vi "OpticsTest.vi"() -> ()   [LabVIEW 2020]
uses:
  opticstest.ctl
panel:
  in  "Case Constant\n(See Context Help)":enum16{"default"}(ring)
  in  "Boolean":bool
  in  "SeqMoveOn":bool
  in  "MoveOn":bool
  out "Options":enum16{"SequenceShot", "SingleShot", "default"}(ring)
  in  "seq":bool
  in  "single":bool
  out "State":enum16{"init", "standby", "loopy", "out"}(ring)
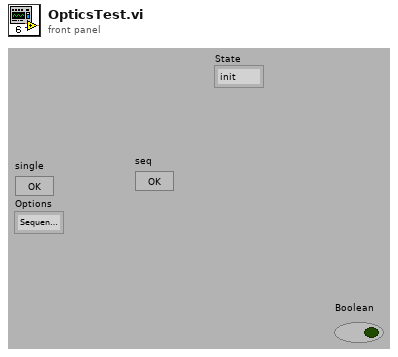
[diagram p1: front panel]
types:
  T1 = typedef "opticstest.ctl" = enum16{"_Quit_", "Init", "Ready", "CCD_shot", "HTL"}
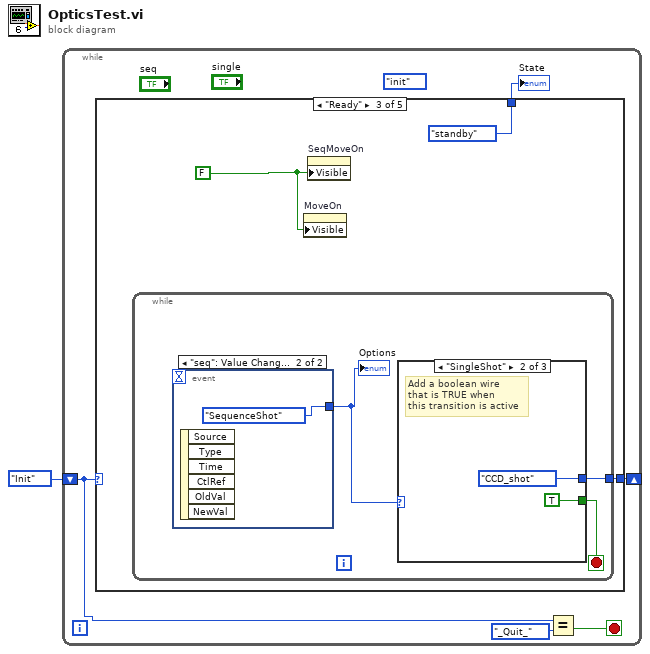
[diagram p0: block diagram]
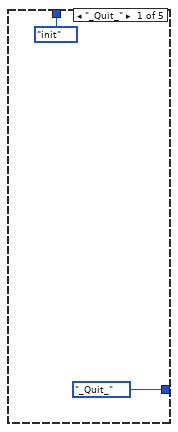
[diagram p2: hidden frame]
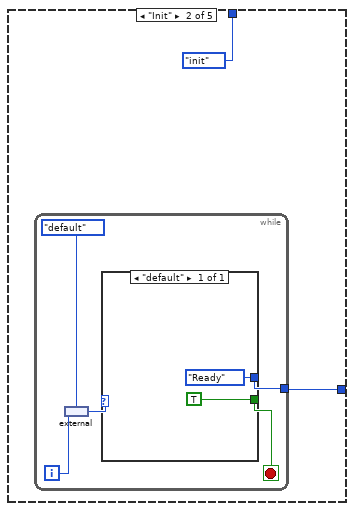
[diagram p3: hidden frame]
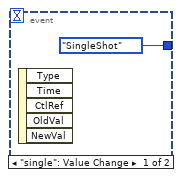
[diagram p4: hidden frame]
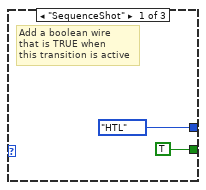
[diagram p5: hidden frame]
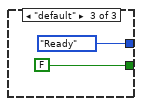
[diagram p6: hidden frame]
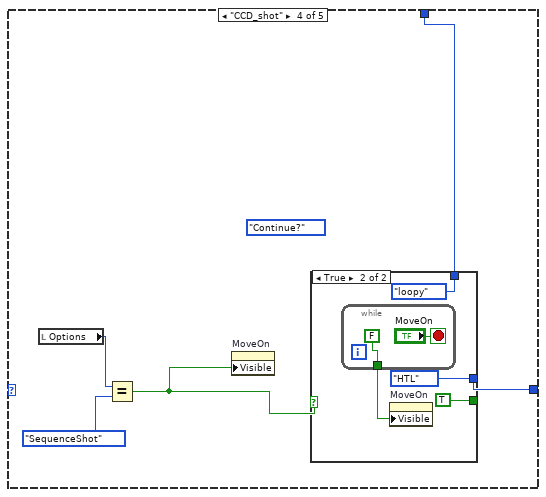
[diagram p7: hidden frame]
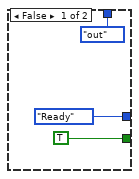
[diagram p8: hidden frame]
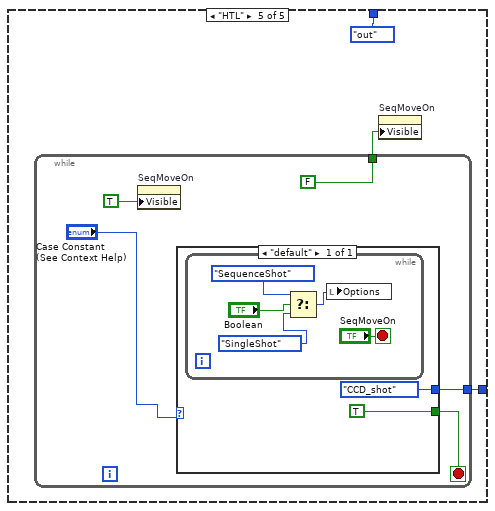
[diagram p9: hidden frame]
diagram:
  n1 = while {
    shift-right: [w5] -> _
    shift-left: opticstest."Init" -> [w6]
    stop <- w4 stop-if-true
    (unwired) enum16{"init", "standby", "loopy", "out"}."init" ("State")
    n2 = case shown="\"Ready\"" w6 {
      tunnel: [opticstest."_Quit_" w10 w25 w41 w53] -> w5
      tunnel: [enum16{"init", "standby", "loopy", "out"}."init" ("State") enum16{"init", "standby", "loopy", "out"}."init" ("State") enum16{"init", "standby", "loopy", "out"}."standby" ("State") w38 enum16{"init", "standby", "loopy", "out"}."out" ("State")] -> w2
      frame "_Quit_" {
      }
      frame "Init" {
        n3 = while {
          tunnel: [w12] -> w10
          i -> [w15]
          stop <- w11 stop-if-true
          n4 = external(enum16{"default"}."default", w15) -> (w13:enum16{"default"})
          n5 = case shown="\"default\"" w13 {
            tunnel: [opticstest."Ready"] -> w12
            tunnel: [TRUE] -> w11
            frame "default" {
            }
          }
        }
      }
      frame "Ready" {
        w23 = FALSE ("Visible")
        n6 = while {
          tunnel: [w28] -> w25
          stop <- w27 stop-if-true
          n7 = event shown="[1] \"seq\": Value Change" {
            selector: _ -> [_ _]
            dyn-events: _ -> [_ _]
            timeout: _ -> [_ _]
            tunnel: [enum16{"SequenceShot", "SingleShot", "default"}."SingleShot" enum16{"SequenceShot", "SingleShot", "default"}."SequenceShot"] -> w26
            event "single": Value Change {
              n8 = event-data() -> ()  [unwired: 1 in, 5 out]
            }
            event "seq": Value Change {
              n9 = event-data() -> ()  [unwired: 1 in, 6 out]
            }
          }
          "Options" <- w26
          n10 = case shown="\"SingleShot\"" w26 {
            tunnel: [opticstest."HTL" opticstest."CCD_shot" opticstest."Ready"] -> w28
            tunnel: [TRUE TRUE FALSE] -> w27
            frame "SequenceShot" {
              # "Add a boolean wire\nthat is TRUE when\nthis transition is active"
            }
            frame "SingleShot" {
              # "Add a boolean wire\nthat is TRUE when\nthis transition is active"
            }
            frame "default" {
            }
          }
        }
        n11 = property on="MoveOn" class="Bool"("Visible"=w23) -> ()  [unwired: 2 in, 2 out]
        n12 = property on="SeqMoveOn" class="Bool"("Visible"=w23) -> ()  [unwired: 2 in, 2 out]
      }
      frame "CCD_shot" {
        (unwired) enum16{"Continue?", "default"}."Continue?"
        n13 = local read "Options"() -> (w40:enum16{"SequenceShot", "SingleShot", "default"})
        n14 = Equal?(x=w40, y=enum16{"SequenceShot", "SingleShot", "default"}."SequenceShot") -> (x = y?=w37:bool)
        n15 = property on="MoveOn" class="Bool"("Visible"=w37) -> ()  [unwired: 2 in, 2 out]
        n16 = case shown="True" w37 {
          tunnel: [opticstest."Ready" opticstest."HTL"] -> w41
          tunnel: [TRUE TRUE] -> _
          tunnel: [enum16{"init", "standby", "loopy", "out"}."out" ("State") enum16{"init", "standby", "loopy", "out"}."loopy" ("State")] -> w38
          frame False {
          }
          frame True {
            n17 = while {
              tunnel: [FALSE ("Visible")] -> w45
              stop <- "MoveOn" stop-if-true
            }
            n18 = property on="MoveOn" class="Bool"("Visible"=w45) -> ()  [unwired: 2 in, 2 out]
          }
        }
      }
      frame "HTL" {
        n19 = while {
          tunnel: [w58] -> w53
          tunnel: [FALSE ("Visible")] -> w51
          stop <- w57 stop-if-true
          n20 = property on="SeqMoveOn" class="Bool"("Visible"=TRUE) -> ()  [unwired: 2 in, 2 out]
          n21 = case shown="\"default\"" "Case Constant\n(See Context Help)" {
            tunnel: [opticstest."CCD_shot"] -> w58
            tunnel: [TRUE] -> w57
            frame "default" {
              n22 = while {
                stop <- "SeqMoveOn" stop-if-true
                n23 = Select(t=enum16{"SequenceShot", "SingleShot", "default"}."SequenceShot" ("Options"), s="Boolean", f=enum16{"SequenceShot", "SingleShot", "default"}."SingleShot" ("Options")) -> (s? t:f=w63:enum16{"SequenceShot", "SingleShot", "default"})
                n24 = local write "Options"(w63) -> ()
              }
            }
          }
        }
        n25 = property on="SeqMoveOn" class="Bool"("Visible"=w51) -> ()  [unwired: 2 in, 2 out]
      }
    }
    "State" <- w2
    n26 = Equal?(x=w6, y=opticstest."_Quit_") -> (x = y?=w4:bool)
  }
